vi "Sort.vi"(11 "TypedCircularBuffer in":refnum<class "VarCircularBuffer.lvclass">) -> (3 "TypedCircularBuffer out":refnum<class "VarCircularBuffer.lvclass">)   [LabVIEW 2024, in "VarCircularBuffer.lvclass"]
uses:
  VarCircularBuffer.lvclass
  VarCircularBuffer.lvclass/VarCircularBuffer.ctl
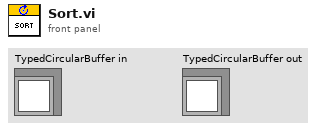
[diagram p1: front panel]
types:
  T1 = typedef "VarCircularBuffer.lvclass/Type.ctl" = i32
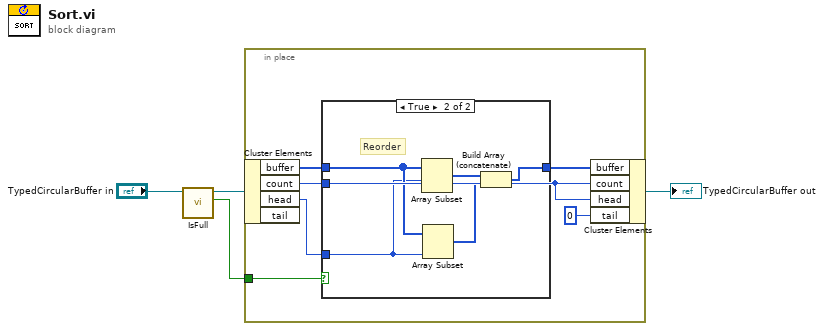
[diagram p0: block diagram]
diagram:
  n1 = call "IsFull.vi"("TypedCircularBuffer in"="TypedCircularBuffer in") -> ("Full?"=w1:bool, "TypedCircularBuffer out"=w2:refnum<class "VarCircularBuffer.lvclass">)  [unwired: 9 in]
  n2 = in-place {
    in-place-border: w1 -> [w5]
    n3 = in-place-cluster #1(w2) -> ("buffer"=w10:T1[], "count"=w6:u32, "head"=w8:u32)  [unwired: 1 out]
    n4 = case shown="True" w5 {
      tunnel: w10 -> [w11 w15]
      tunnel: [w11 w16] -> w9
      tunnel: w6 -> [_ _]
      tunnel: w8 -> [_ w14]
      frame False {
      }
      frame True {
        # "Reorder"
        n5 = Array Subset(array=w15, index=w14) -> (w13:T1[])  [unwired: 1 in]
        n6 = Array Subset(array=w15, length=w14) -> (w12:T1[])  [unwired: 1 in]
        n7 = Build Array (concatenate)(w13, w12) -> (w16:T1[])
      }
    }
    n8 = in-place-cluster #1("buffer"=w9, "count"=w6, "head"=w6, "tail"=u32 0 ("head")) -> (→"TypedCircularBuffer out":refnum<class "VarCircularBuffer.lvclass">)
  }
